vi "Update Selector Channel.vi"(8 "error in":errorcluster, 10 "Global Selector":bool, 11 "Node Ptr":T1 format="%.0x") -> (0 "error out":errorcluster)   [LabVIEW 2021, in "Software Multi-Plex System Explorer.lvlib"]
uses:
  Software Multi-Plex System Explorer.lvlib
  <vilib>/NI VeriStand/Custom Device API/Custom Device Item Ref.ctl
  <vilib>/NI VeriStand/Custom Device API/Custom Device Channel.ctl
  <vilib>/NI VeriStand/Custom Device API/Custom Device Channel Type.ctl
  Shared/Constants.vi
  <vilib>/NI VeriStand/Custom Device Tools/Custom Device Utility Library/NI VeriStand - Search for All Items by GUID.vi
  <vilib>/NI VeriStand/Custom Device Tools/Custom Device Utility Library/Custom Device Utility Library.lvlib
  Shared/Software Multi-Plex Shared.lvlib
  <vilib>/NI VeriStand/Custom Device API/Custom Device API.lvlib
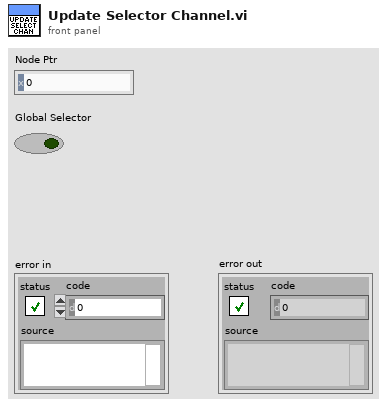
[diagram p1: front panel]
types:
  T1 = typedef "Custom Device API.lvlib/Custom Device Item Ref.ctl" = u64
  T2 = typedef "Custom Device API.lvlib/Custom Device Channel.ctl" = cluster{"Type":T3, "Units":string, "Default Value":dbl, "Faultable":bool, "Scalable":bool}
  T3 = typedef "Custom Device API.lvlib/Custom Device Channel Type.ctl" = enum16{"Input", "Output"}
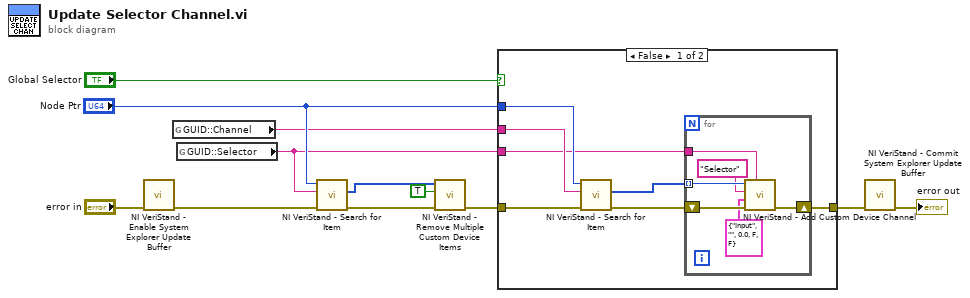
[diagram p0: block diagram]
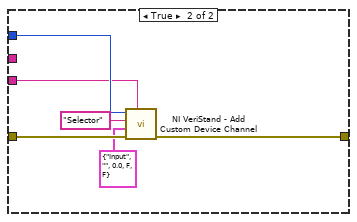
[diagram p2: hidden frame]
diagram:
  n1 = call <vilib>:"NI VeriStand - Enable System Explorer Update Buffer.vi"("error in (no error)"="error in") -> ("error out"=w8:errorcluster)  [unwired: 10 in]
  n2 = global read "Constants.vi" "GUID::Channel"() -> (w2:string)
  n3 = global read "Constants.vi" "GUID::Selector"() -> (w4:string)
  n4 = call-poly <vilib>:"NI VeriStand - Search for Item.vi"("error in"=w8, "Item GUID"=w4, "Section Ref in"="Node Ptr") -> ("error out"=w12:errorcluster, "Item Refs"=w11:T1[])  [unwired: 5 in, 2 out]
  n5 = call <vilib>:"NI VeriStand - Remove Multiple Custom Device Items.vi"("error in (no error)"=w12, "Force Delete (F)"=TRUE, "Item Refs in"=w11) -> ("error out"=w7:errorcluster)  [unwired: 7 in, 1 out]
  n6 = case shown="False" "Global Selector" {
    tunnel: w7 -> [w19 w31]
    tunnel: "Node Ptr" -> [w18 w30]
    tunnel: w4 -> [w14 w27]
    tunnel: [w13 w26] -> w3
    tunnel: w2 -> [w17 _]
    frame False {
      n7 = call-poly <vilib>:"NI VeriStand - Search for Item.vi"("error in"=w19, "Item GUID"=w17, "Section Ref in"=w18) -> ("error out"=w16:errorcluster, "Item Refs"=w15:T1[])  [unwired: 5 in, 2 out]
      n8 = for {
        shift-right: [w24] -> w13
        shift-left: w16 -> [w25]
        tunnel: w15 -> [w23] mode=indexing
        tunnel: w14 -> [w22]
        n9 = call <vilib>:"NI VeriStand - Add Custom Device Channel.vi"("GUID (Default Channel)"=w22, "error in (no error)"=w25, "Channel"=T2 {"Type"=enum."Input", "Units"="", "Default Value"=0.0, "Faultable"=FALSE, "Scalable"=FALSE}, "Channel Name"="Selector", "Parent Ref in"=w23) -> ("error out"=w24:errorcluster)  [unwired: 3 in, 3 out]
      }
    }
    frame True {
      n10 = call <vilib>:"NI VeriStand - Add Custom Device Channel.vi"("GUID (Default Channel)"=w27, "error in (no error)"=w31, "Channel"=T2 {"Type"=enum."Input", "Units"="", "Default Value"=0.0, "Faultable"=FALSE, "Scalable"=FALSE}, "Channel Name"="Selector", "Parent Ref in"=w30) -> ("error out"=w26:errorcluster)  [unwired: 3 in, 3 out]
    }
  }
  n11 = call <vilib>:"NI VeriStand - Commit System Explorer Update Buffer.vi"("error in (no error)"=w3) -> ("error out"=→"error out":errorcluster)  [unwired: 10 in]
